vi "App.Initialize.vi"(8 "error in (no error)":errorcluster, 11 "Start Variables":T1={"Aliases.All"=[], "Aliases.Outputs"=[], "UI.Sequence#ofColumns"=0, "SysDef.Path"=path "", "UI.SequenceRef"=refnum, "UI.StepInformationRef"=refnum, "UI.AbortRef"=refnum, "UI.GraphRef"=refnum, "UI.ViewRef"=refnum, "UI.IterationsRef"=refnum, "UI.IterationInformationRef"=refnum, "INI.Settings"={"Build Location"=path "C:/Simple Sequence Editor/SequenceRepo", "LoggingLocation"=path ""}, "NIVS.Workspace Event"=refnum, "UI.SkipChannel"=refnum, "NIVS.Launched?"=FALSE, "UI.DurationChannel"=refnum}) -> (0 "error out":errorcluster)   [LabVIEW 2015, in "Simple Sequence Tools - Editor.lvlib"]
uses:
  Simple Sequence Tools - Editor.lvlib
  Types/Main.StateVariables.ctl
  Shared/Types/Channel.Properties.ctl
  Shared/Types/INI.Settings
  Types/UI.PropertiesTypes.ctl
  Shared/SubVIs/Main.Constants.vi
  Shared/Simple Sequence Tools - Shared.lvlib
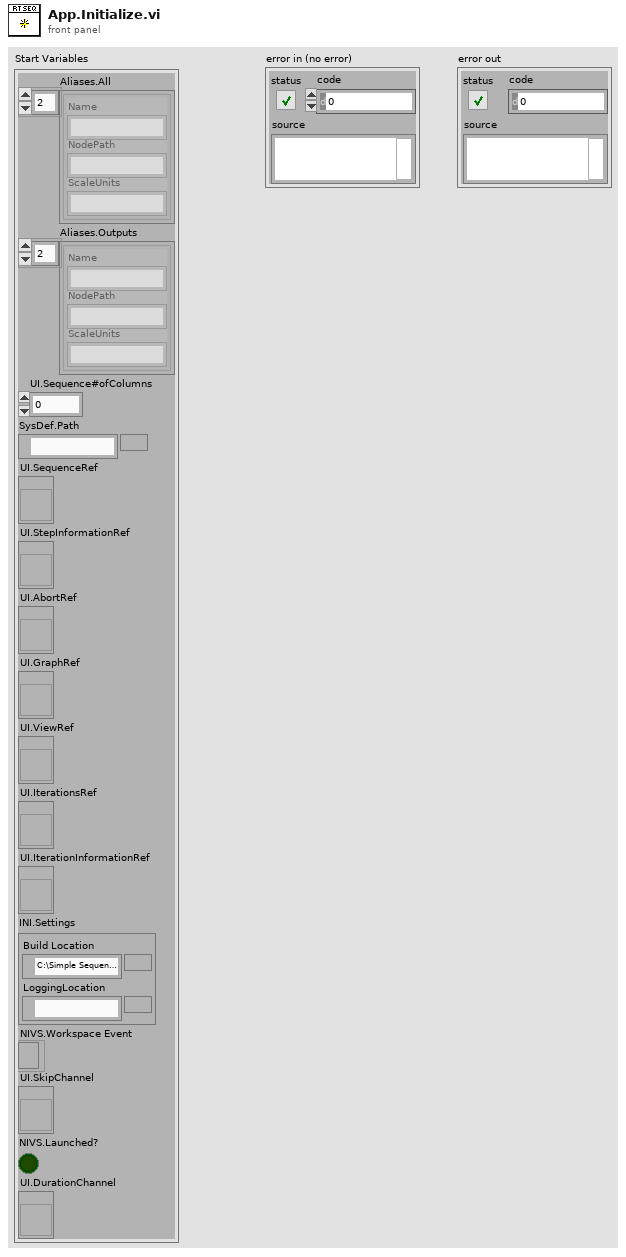
[diagram p1: front panel]
types:
  T1 = typedef "Simple Sequence Tools - Editor.lvlib/Main.StateVariables.ctl" = cluster{"Aliases.All":T2[], "Aliases.Outputs":T2[], "UI.Sequence#ofColumns":i32, "SysDef.Path":path, "UI.SequenceRef":refnum<vi>, "UI.StepInformationRef":refnum<vi>, "UI.AbortRef":refnum<vi>, "UI.GraphRef":refnum<vi>, "UI.ViewRef":refnum<vi>, "UI.IterationsRef":refnum<vi>, "UI.IterationInformationRef":refnum<vi>, "INI.Settings":T3, "NIVS.Workspace Event":refnum<event-registration>, "UI.SkipChannel":refnum<vi>, "NIVS.Launched?":bool, "UI.DurationChannel":refnum<vi>}
  T2 = typedef "Simple Sequence Tools - Shared.lvlib/Channel.Properties.ctl" = cluster{"Name":string, "NodePath":string, "ScaleUnits":string}
  T3 = typedef "Simple Sequence Tools - Shared.lvlib/INI.Settings" = cluster{"Build Location":path, "LoggingLocation":path}
  T4 = typedef "Simple Sequence Tools - Editor.lvlib/UI.PropertiesTypes.ctl" = enum8{"Step Properties", "Sequence Properties"}
  T5 = typedef "LVBoundsTypeDef.ctl" = cluster{"Width":u32, "Height":u32}
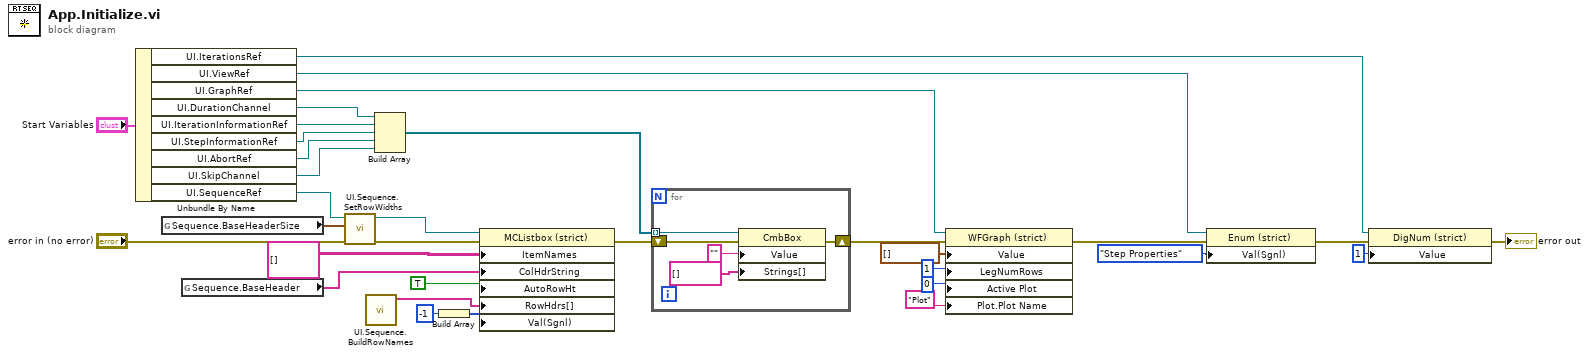
[diagram p0: block diagram]
diagram:
  n1 = Unbundle By Name("Start Variables") -> ("UI.IterationsRef"=w7:refnum<vi>, "UI.ViewRef"=w29:refnum<vi>, "UI.GraphRef"=w23:refnum<vi>, "UI.DurationChannel"=w1:refnum<vi>, "UI.IterationInformationRef"=w3:refnum<vi>, "UI.StepInformationRef"=w21:refnum<vi>, "UI.AbortRef"=w20:refnum<vi>, "UI.SkipChannel"=w2:refnum<vi>, "UI.SequenceRef"=w15:refnum<vi>)
  n2 = global read "Main.Constants.vi" "Sequence.BaseHeaderSize"() -> (w8:T5[])
  n3 = global read "Main.Constants.vi" "Sequence.BaseHeader"() -> (w9:string[])
  n4 = call "UI.Sequence.SetRowWidths.vi"("error in (no error)"="error in (no error)", "CellSize"=w8, "UI.SequenceRef"=w15) -> ("error out"=w14:errorcluster, "UI.SequenceRef"=w16:refnum<vi>)  [unwired: 7 in]
  n5 = call "UI.Sequence.BuildRowNames.vi"() -> ("Row Headings"=w17:string[])  [unwired: 11 in]
  n6 = Build Array(w1, w3, w21, w20, w2) -> (w22:refnum<vi>[])
  n7 = Build Array(-1 ("Value")) -> (w19:i32[])
  n8 = property class="MCListbox (strict)"(reference=w16, error in=w14, "ItemNames"=string[][] [] ("Item Names"), "ColHdrString"=w9, "AutoRowHt"=TRUE ("Autosizing Row Height"), "RowHdrs[]"=w17, "Val(Sgnl)"=w19) -> (error out=w32:errorcluster)  [unwired: 1 out]
  n9 = for {
    tunnel: w22 -> [w36] mode=indexing
    shift-right: [w34] -> w24
    shift-left: w32 -> [w37]
    n10 = property class="CmbBox"(reference=w36, error in=w37, "Value"="", "Strings[]"=string[] [] ("Strings []")) -> (error out=w34:errorcluster)  [unwired: 1 out]
  }
  n11 = property class="WFGraph (strict)"(reference=w23, error in=w24, "Value"=waveform(dbl)[] [], "LegNumRows"=u32 1 ("Legend:Number of Rows"), "Active Plot"=u32 0, "Plot.Plot Name"="Plot") -> (error out=w30:errorcluster)  [unwired: 1 out]
  n12 = property class="Enum (strict)"(reference=w29, error in=w30, "Val(Sgnl)"=UI.PropertiesTypes."Step Properties" ("Value (Signaling)")) -> (error out=w6:errorcluster)  [unwired: 1 out]
  n13 = property class="DigNum (strict)"(reference=w7, error in=w6, "Value"=u32 1) -> (error out=→"error out":errorcluster)  [unwired: 1 out]
